vi "build_path_by_string.vi"() -> ()   [LabVIEW 2025]
uses:
  <vilib>/Utility/sysdir.llb/System Directory Type.ctl
panel:
  out "appended path":path
  in  "base path":path
  in  "String":string
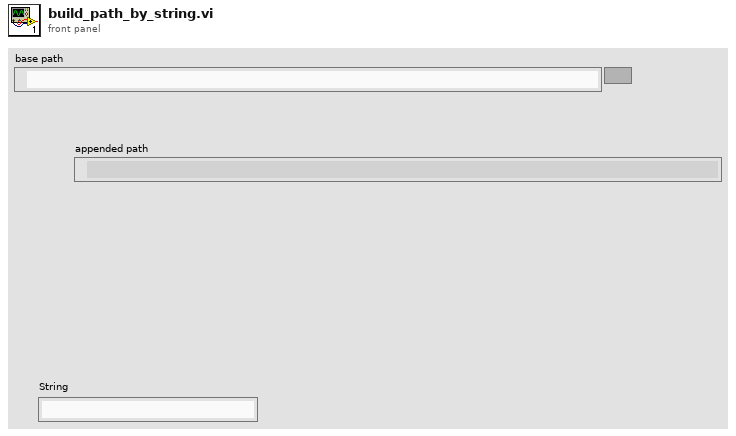
[diagram p1: front panel]
types:
  T1 = typedef "System Directory Type.ctl" = i32
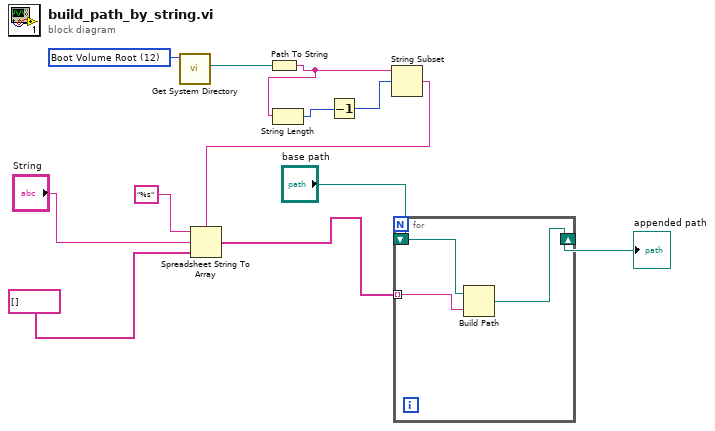
[diagram p0: block diagram]
diagram:
  w10 = T1 12 items=["User Home"=0, "User Desktop"=1, "User Documents"=2, "User Application Data"=3, "User Preferences"=4, "User Temporary"=5, "Public Documents"=6, "Public Application Data"=7, "Public Preferences"=8, "Public Cache"=13, "System Core Libraries"=9, "System Installed Libraries"=10, "Application Files"=11, "Boot Volume Root"=12] ("system directory type")
  n1 = call <vilib>:"Get System Directory.vi"("system directory type"=w10) -> ("system directory"=w1:path)  [unwired: 10 in]
  n2 = Path To String(path=w1) -> (string=w9:string)
  n3 = String Length(string=w9) -> (length=w8:i32)
  n4 = Decrement(x=w8) -> (x-1=w7:i32)
  n5 = String Subset(string=w9, offset (0)=w7) -> (substring=w6:string)  [unwired: 1 in]
  n6 = Spreadsheet String To Array(delimiter (Tab)=w6, format string="%s", spreadsheet string="String", array type (2D Dbl)=string[] [] ("Array 2")) -> (array=w2:string[])
  n7 = for {
    shift-right: [w14] -> w4
    shift-left: "base path" -> [w15]
    tunnel: w2 -> [w13] mode=indexing
    n8 = Build Path(base path=w15, name or relative path=w13) -> (appended path=w14:path)
  }
  "appended path" <- w4
